vi "Initialize.vi"(8 "error in (no error)":errorcluster) -> (0 "error out":errorcluster)   [LabVIEW 2020, in "CodeSignAPI.lvlib"]
doc: "nicsgnInit(void);"
uses:
  <vilib>/AppBuilder/CodeSignAPI/CodeSignAPI.lvlib
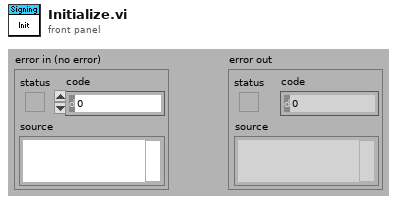
[diagram p1: front panel]
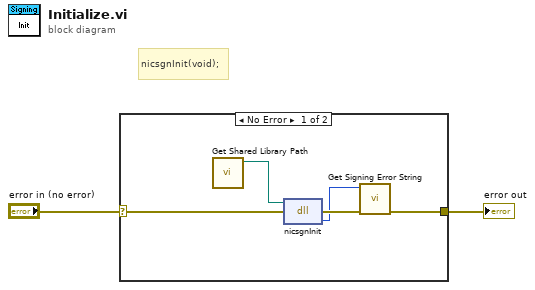
[diagram p0: block diagram]
diagram:
  # "nicsgnInit(void);"
  n1 = case shown="No Error" "error in (no error)" {
    selector: "error in (no error)" -> [w6 w8]
    tunnel: [w5 w8] -> w2
    frame No Error {
      n2 = call <vilib>:"Get Shared Library Path.vi"() -> ("shared library path"=w7:path)  [unwired: 1 in, 10 out]
      n3 = dll-call lib="?" fn="nicsgnInit"(path in=w7, error in=w6) -> (error out=w4:errorcluster, "return type"=w3:i64)  [unwired: 1 in, 1 out]
      n4 = call <vilib>:"Get Signing Error String.vi"("error in (no error)"=w4, "NICSGN_ERROR"=w3) -> ("error out"=w5:errorcluster)  [unwired: 9 out]
    }
    frame Error {
    }
  }
  "error out" <- w2
